vi "RegisterToAckMessage.vi"(8 "error in (no error)":errorcluster, 9 "explicit acknowledgement":bool=TRUE, 10 "message name":string, 11 "subscriber in":refnum<class "IcmMessageSubscriber.lvclass">) -> (0 "error out":errorcluster, 3 "subscriber out":refnum<class "IcmMessageSubscriber.lvclass">)   [LabVIEW 2017, in "IcmMessageSubscriber.lvclass"]
doc: "Registers a message to require explicit acknowledgement."
uses:
  <vilib>/addons/InsightCM/MessageBus/MessageSubscriber/IcmMessageSubscriber.lvclass
  <vilib>/addons/InsightCM/MessageBus/MessageSubscriber/IcmMessageSubscriber.lvclass/IcmMessageSubscriber.ctl
  C:/Program Files (x86)/National Instruments/LabVIEW 2017/vi.lib/addons/InsightCM/Binaries/LabviewMessageAdapter.dll
  Binaries/LabviewMessageAdapter.dll
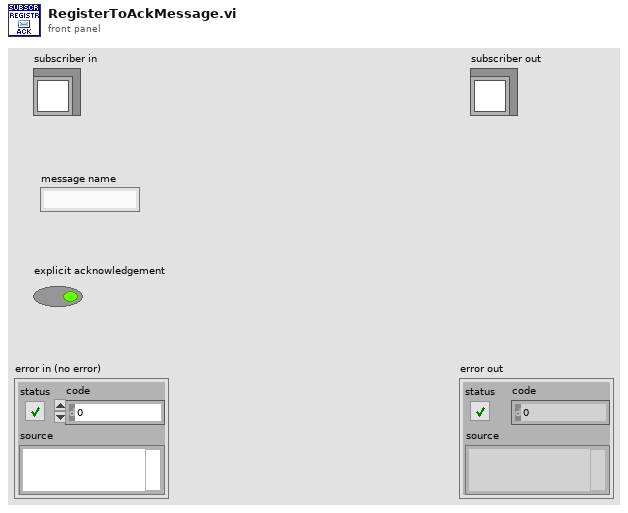
[diagram p1: front panel]
types:
  T1 = typedef "MessageSubscriberDvr.ctl" = refnum<data-value>
  T2 = typedef "MessageSubscriberData.ctl" = cluster{"Subscriber":refnum<k24>}
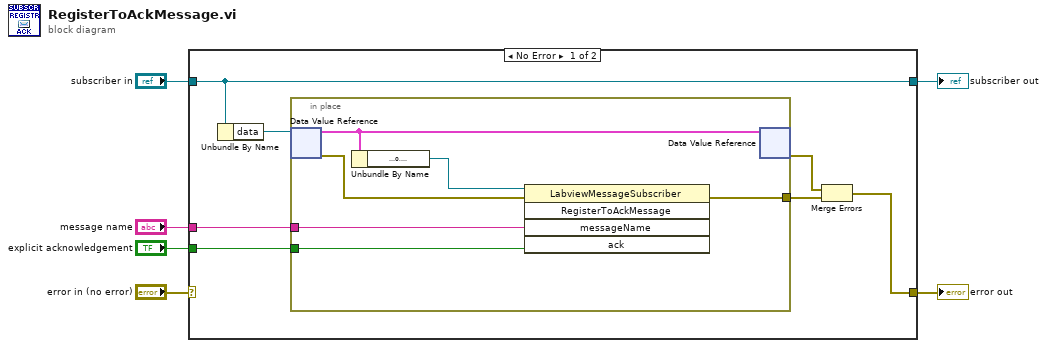
[diagram p0: block diagram]
diagram:
  n1 = case shown="No Error" "error in (no error)" {
    selector: "error in (no error)" -> [_ w21]
    tunnel: [w9 w21] -> w5
    tunnel: "subscriber in" -> [w8 w20]
    tunnel: "message name" -> [w10 _]
    tunnel: [w8 w20] -> w3
    tunnel: "explicit acknowledgement" -> [w7 _]
    frame No Error {
      n2 = Unbundle By Name(w8) -> ("data"=w13:T1)
      n3 = in-place {
        in-place-border: [w18] -> w11
        in-place-border: w10 -> [w15]
        in-place-border: w7 -> [w14]
        n4 = in-place-dvr #1(w13) -> (w19:T2, w17:errorcluster)
        n5 = Unbundle By Name(w19) -> ("Subscriber"=w16:refnum<k24>)
        n6 = invoke class="LabviewMessageSubscriber" method="RegisterToAckMessage"(reference=w16, error in=w17, "messageName"=w15, "ack"=w14) -> (error out=w18:errorcluster)  [unwired: 1 in, 4 out]
        n7 = in-place-dvr #1(w19) -> (w12:errorcluster)  [unwired: 1 out]
      }
      n8 = Merge Errors(w12, w11) -> (w9:errorcluster)
    }
    frame Error {
    }
  }
  "error out" <- w5
  "subscriber out" <- w3
